vi "Print Buffer Data.vi"(7 "Reading Buffer (smua.nvbuffer1)":string="smua.nvbuffer1", 8 "error in (no error)":errorcluster, 9 "End Index (1)":i32=1, 10 "Start Index (1)":i32=1, 11 "VISA resource name":refnum<visa-resource-name>) -> (0 "error out":errorcluster, 2 "Buffer Data":dbl[](array[numeric]), 3 "VISA resource name out":refnum<visa-resource-name>)   [LabVIEW 2020, in "Keithley 2600 Series.lvlib"]
doc: "Prints data from tables or reading buffer sub-tables."
uses:
  Keithley 2600 Series.lvlib
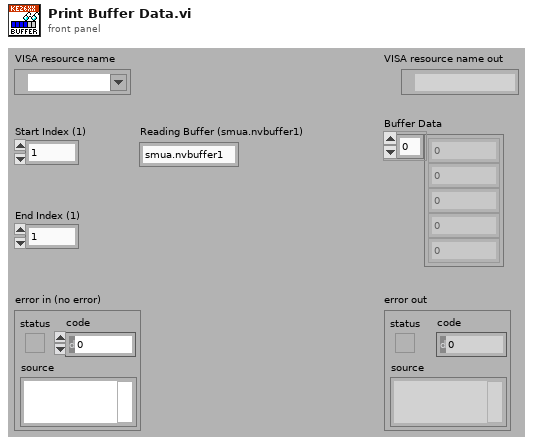
[diagram p1: front panel]
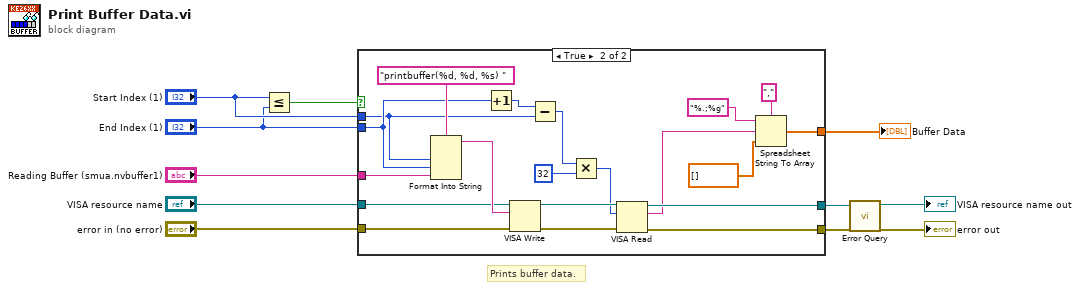
[diagram p0: block diagram]
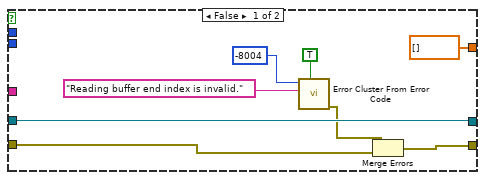
[diagram p2: hidden frame]
diagram:
  # "Prints buffer data."
  n1 = Less Or Equal?(x="Start Index (1)", y="End Index (1)") -> (x <= y?=w1:bool)
  n2 = case shown="True" w1 {
    tunnel: "Start Index (1)" -> [_ w21]
    tunnel: "End Index (1)" -> [_ w22]
    tunnel: "Reading Buffer (smua.nvbuffer1)" -> [_ w38]
    tunnel: "VISA resource name" -> [w19 w36]
    tunnel: "error in (no error)" -> [w12 w35]
    tunnel: [w19 w33] -> w6
    tunnel: [w17 w31] -> w5
    tunnel: [dbl[] [] ("array type (2D Dbl)") w26] -> w4
    frame False {
      n3 = call <vilib>:"Error Cluster From Error Code.vi"("show call chain? (False)"=TRUE, "error message (\"\")"="Reading buffer end index is invalid." ("error message (\"\")"), "error code (0)"=-8004) -> ("error out"=w13:errorcluster)  [unwired: 6 in]
      n4 = Merge Errors(w13, w12) -> (w17:errorcluster)
    }
    frame True {
      n5 = Format Into String(format string="printbuffer(%d, %d, %s) ", w21, w22, w38) -> (resulting string=w37:string)  [unwired: 2 in, 1 out]
      n6 = Increment(x=w22) -> (x+1=w20:i32)
      n7 = VISA Write(VISA resource name=w36, write buffer=w37, error in (no error)=w35) -> (VISA resource name out=w34:refnum<visa-resource-name>, error out=w32:errorcluster)  [unwired: 1 out]
      n8 = Subtract(x=w20, y=w21) -> (x-y=w25:i32)
      n9 = Multiply(x=w25, y=32) -> (x*y=w24:i32)
      n10 = VISA Read(VISA resource name=w34, byte count=w24, error in (no error)=w32) -> (VISA resource name out=w33:refnum<visa-resource-name>, read buffer=w30:string, error out=w31:errorcluster)  [unwired: 1 out]
      n11 = Spreadsheet String To Array(delimiter (Tab)=",", format string="%.;%g", spreadsheet string=w30, array type (2D Dbl)=dbl[] []) -> (array=w26:dbl[])
    }
  }
  "Buffer Data" <- w4
  n12 = call "Error Query.vi"("error in (no error)"=w5, "VISA resource name"=w6) -> ("error out"=→"error out":errorcluster, "VISA resource name out"=→"VISA resource name out":refnum<visa-resource-name>)  [unwired: 6 in, 2 out]
